vi "File_Create Linker files.vi"(7 "Run Data":T1={"Target Folder"=path "", "Menu Folder"=path "", "Active Folder"=path "", "Config"={"Main"={"Menu Folder"="", "Re-Create Menu Folder?"=FALSE, "Allow mnu replace?"=FALSE, "Relative Link Target"=""}, "File Filter"={"Exclude Prefixes"=[], "Ignore Names"=[], "Include Extensions"=[], "Exclude Postfixes"=[]}, "Folder Filter"={"Exclude Prefixes"=[], "Ignore Names"=[]}, "File Name Edit"={"Pre Split String"="", "Post Split String"="", "Deletion Strings"=[]}, "Folder Name Edit"={"Pre Split String"="", "Post Split String"="", "Deletion Strings"=[]}, "Folder Icon Map"={}, "Default Palette Data"={"Display Name Override"="", "View Format"=2, "Palette Width"=0, "Help Tag"="", "Help File Path"=path "", "Palette Description"=""}, "Default File Data"={"Display Name Override"="", "Place VI Contents?"=FALSE}, "Palette Override map"={}, "File Override map"={}}} {"Config"."Default Palette Data"."View Format" items=["Icons", "Text", "Icons and Text"]}, 8 "error in (no error)":errorcluster, 10 "Link Target Root Override (\"\")":path, 11 "Created mnu file paths":path[](array[path])) -> (0 "error out":errorcluster, 1 "Link files created?":bool, 2 "Unlinker":path, 3 "Linker":path)   [LabVIEW 2019, in "AutoMenuCreator.lvlib"]
uses:
  AutoMenuCreator.lvlib
  Ctl/Ctl_Run Data.ctl
  Ctl/Ctl_Config.ctl
  Ctl/Ctl_Config_Main.ctl
  Ctl/Ctl_Config_File Filter.ctl
  Ctl/Ctl_Config_Folder Filter.ctl
  Ctl/Ctl_Config_Name Edit.ctl
  Ctl/Ctl_Config_Folder Icon Map.ctl
  Ctl/Ctl_Config_Palette Data.ctl
  <vilib>/Palette API/Palette Menu/Public Type Define/View Format.ctl
  Ctl/Ctl_Config_File Data.ctl
  <vilib>/Palette API/Palette Menu/Palette Menu.lvlib
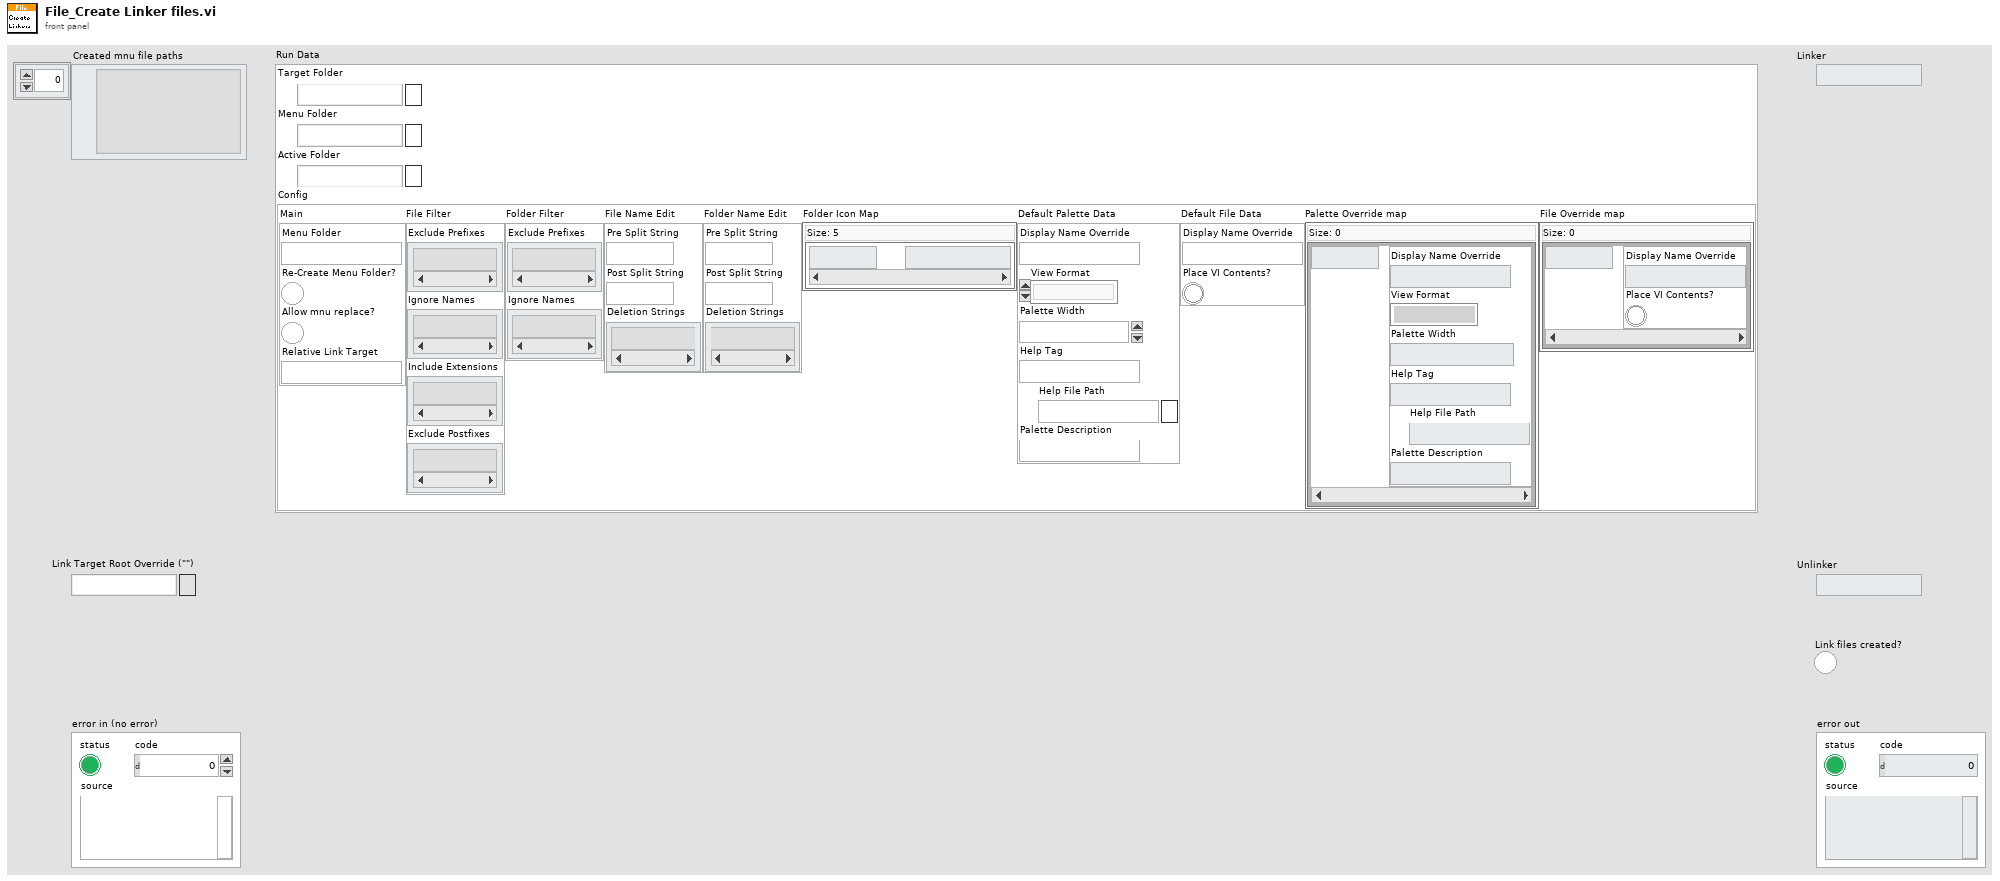
[diagram p1: front panel]
types:
  T1 = typedef "AutoMenuCreator.lvlib/Ctl_Run Data.ctl" = cluster{"Target Folder":path, "Menu Folder":path, "Active Folder":path, "Config":T2}
  T2 = typedef "AutoMenuCreator.lvlib/Ctl_Config.ctl" = cluster{"Main":T3, "File Filter":T4, "Folder Filter":T5, "File Name Edit":T6, "Folder Name Edit":T6, "Folder Icon Map":T7, "Default Palette Data":T8, "Default File Data":T10, "Palette Override map":map{string, T8}, "File Override map":map{string, T10}}
  T3 = typedef "AutoMenuCreator.lvlib/Ctl_Config_Main.ctl" = cluster{"Menu Folder":string, "Re-Create Menu Folder?":bool, "Allow mnu replace?":bool, "Relative Link Target":string}
  T4 = typedef "AutoMenuCreator.lvlib/Ctl_Config_File Filter.ctl" = cluster{"Exclude Prefixes":string[], "Ignore Names":string[], "Include Extensions":string[], "Exclude Postfixes":string[]}
  T5 = typedef "AutoMenuCreator.lvlib/Ctl_Config_Folder Filter.ctl" = cluster{"Exclude Prefixes":string[], "Ignore Names":string[]}
  T6 = typedef "AutoMenuCreator.lvlib/Ctl_Config_Name Edit.ctl" = cluster{"Pre Split String":string, "Post Split String":string, "Deletion Strings":string[]}
  T7 = typedef "AutoMenuCreator.lvlib/Ctl_Config_Folder Icon Map.ctl" = map{string, path}
  T8 = typedef "AutoMenuCreator.lvlib/Ctl_Config_Palette Data.ctl" = cluster{"Display Name Override":string, "View Format":T9, "Palette Width":i16, "Help Tag":string, "Help File Path":path, "Palette Description":string}
  T9 = typedef "Palette Menu.lvlib/View Format.ctl" = u16
  T10 = typedef "AutoMenuCreator.lvlib/Ctl_Config_File Data.ctl" = cluster{"Display Name Override":string, "Place VI Contents?":bool}
  T11 = enum16{"open", "replace", "create", "open or create", "replace or create", "replace or create with confirmation"}
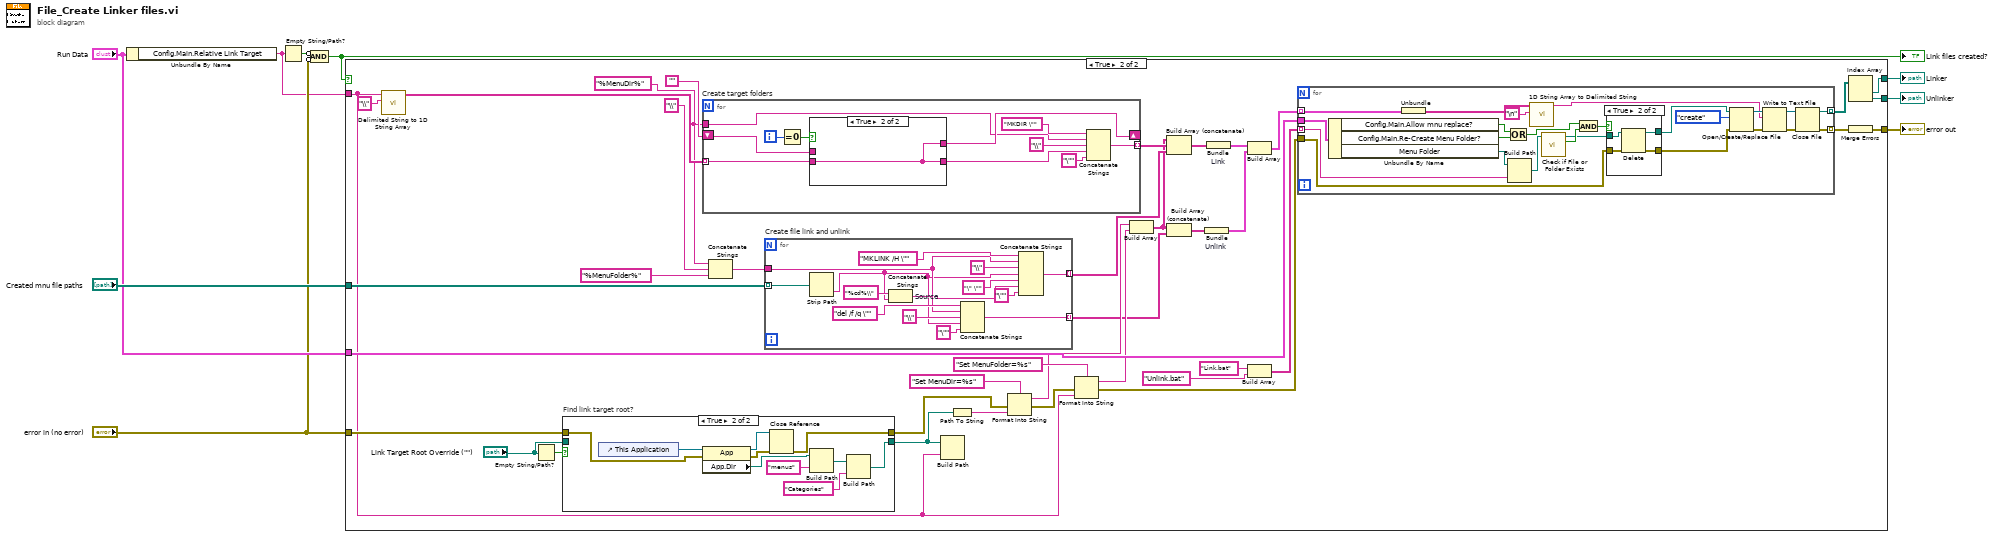
[diagram p0: block diagram]
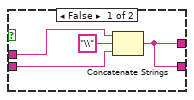
[diagram p4: hidden frame]
diagram:
  n1 = Unbundle By Name("Run Data") -> ("Config.Main.Relative Link Target"=w4:string)
  n2 = Empty String/Path?(string/path=w4) -> (empty?=w7:bool)
  n3 = Compound Arithmetic op=AND(invert w7, invert "error in (no error)") -> (w5:bool)
  "Link files created?" <- w5
  n4 = case shown="True" w5 {
    tunnel: "Created mnu file paths" -> [_ w49]
    tunnel: "Run Data" -> [_ w33]
    tunnel: "error in (no error)" -> [w10 w46]
    tunnel: w4 -> [_ w23]
    tunnel: [w10 w31] -> w3
    tunnel: [_ w29] -> w2
    tunnel: [_ w28] -> w1
    frame False {
    }
    frame True {
      w13 = "%MenuDir%"
      n5 = call <vilib>:"Delimited String to 1D String Array.vi"("delimiter"="\\", "delimited string"=w23) -> ("string array"=w44:string[])  [unwired: 9 in]
      n6 = Empty String/Path?(string/path="Link Target Root Override (\"\")") -> (empty?=w48:bool)
      n7 = case "Find link target root?" shown="True" w48 {
        tunnel: [w97 w100] -> w27
        tunnel: "Link Target Root Override (\"\")" -> [w97 _]
        tunnel: w46 -> [w96 w99]
        tunnel: [w96 w98] -> w21
        frame False {
        }
        frame True {
          n8 = control-ref of="This Application"() -> (w107:refnum<vi>)
          n9 = property class="App"(reference=w107, error in=w99) -> (reference out=w105:refnum<vi>, error out=w106:errorcluster, "App.Dir"=w104:path)
          n10 = Close Reference(reference=w105, error in (no error)=w106) -> (error out=w98:errorcluster)
          n11 = Build Path(base path=w104, name or relative path="menus") -> (appended path=w102:path)
          n12 = Build Path(base path=w102, name or relative path="Categories") -> (appended path=w100:path)
        }
      }
      n13 = for "Create target folders" {
        tunnel: w44 -> [w88] mode=indexing
        shift-right: [w86] -> _
        shift-left: "" -> [w87]
        tunnel: [w80] -> w42 mode=indexing
        tunnel: w13 -> [w84]
        i -> [w90]
        n14 = Equal To 0?(x=w90) -> (x = 0?=w89:bool)
        n15 = case shown="True" w89 {
          tunnel: [w91 w95] -> w82
          tunnel: w88 -> [w92 w95]
          tunnel: w87 -> [w94 _]
          tunnel: [w91 w95] -> w86
          frame False {
            n16 = Concatenate Strings(w94, "\\" ("string"), w92) -> (w91:string)
          }
          frame True {
          }
        }
        n17 = Concatenate Strings("MKDIR \"" ("string"), w84, "\\" ("string"), w82, "\"" ("string")) -> (w80:string)
      }
      n18 = Concatenate Strings(w13, "\\" ("string"), "%MenuFolder%") -> (w19:string)
      n19 = for "Create file link and unlink" {
        tunnel: w49 -> [w121] mode=indexing
        tunnel: [w109] -> w41 mode=indexing
        tunnel: [w116] -> w15 mode=indexing
        tunnel: w19 -> [w114]
        n20 = Strip Path(path=w121) -> (name=w108:string)  [unwired: 1 out]
        n21 = Concatenate Strings "Source"("%cd%\\", w108) -> (w111:string)
        n22 = Concatenate Strings("del /f /q \"" ("string"), w114, "\\" ("string"), w108, "\"" ("string")) -> (w116:string)
        n23 = Concatenate Strings("MKLINK /H \"" ("string"), w114, "\\" ("string"), w108, "\" \"" ("string"), w111, "\"" ("string")) -> (w109:string)
      }
      n24 = Build Path(base path=w27, name or relative path=w23) -> ()  [unwired: 1 out]
      n25 = Path To String(path=w27) -> (string=w25:string)
      n26 = Format Into String(format string="Set MenuDir=%s", error in=w21, w25) -> (resulting string=w18:string, error out=w22:errorcluster)  [unwired: 1 in]
      n27 = Format Into String(format string="Set MenuFolder=%s", error in=w22, w23) -> (resulting string=w17:string, error out=w11:errorcluster)  [unwired: 1 in]
      n28 = Build Array(w18, w17) -> (w16:string[])
      n29 = Build Array (concatenate)(w16, w42, w41) -> (w40:string[])
      n30 = Build Array (concatenate)(w16, w15) -> (w14:string[])
      n31 = Bundle "Unlink"(w14) -> (w38:cluster{string[]})  [unwired: 1 in]
      n32 = Bundle "Link"(w40) -> (w39:cluster{string[]})  [unwired: 1 in]
      n33 = Build Array(w39, w38) -> (w37:cluster{string[]}[])
      n34 = Build Array("Link.bat" ("string"), "Unlink.bat" ("string")) -> (w34:string[])
      n35 = for {
        tunnel: w11 -> [w63]
        tunnel: w37 -> [w73] mode=indexing
        tunnel: w34 -> [w68] mode=indexing
        tunnel: w33 -> [w71]
        tunnel: [w51] -> w32 mode=indexing
        tunnel: [w50] -> w30 mode=indexing
        n36 = Unbundle By Name(w71) -> ("Config.Main.Allow mnu replace?"=w70:bool, "Config.Main.Re-Create Menu Folder?"=w72:bool, "Menu Folder"=w69:path)
        n37 = Unbundle(w73) -> (w58:string[])
        n38 = Or(x=w70, y=w72) -> (x .or. y?=w65:bool)
        n39 = Build Path(base path=w69, name or relative path=w68) -> (appended path=w67:path)
        n40 = call <vilib>:"1D String Array to Delimited String.vi"("delimiter"="\n", "string array"=w58) -> ("delimited string"=w55:string)  [unwired: 9 in]
        n41 = call <vilib>:"Check if File or Folder Exists.vi"("path"=w67) -> ("file or folder exists?"=w66:bool, "dup path"=w62:path)  [unwired: 8 in, 1 out]
        n42 = And(x=w65, y=w66) -> (x .and. y?=w64:bool)
        n43 = case shown="True" w64 {
          tunnel: [w75 w78] -> w59
          tunnel: w63 -> [w75 w79]
          tunnel: w62 -> [w74 w77]
          tunnel: [w74 w76] -> w61
          frame False {
          }
          frame True {
            n44 = Delete(path (use dialog)=w77, error in=w79) -> (deleted path=w76:path, error out=w78:errorcluster)  [unwired: 3 in, 1 out]
          }
        }
        n45 = Open/Create/Replace File(file path (use dialog)=w61, error in=w59, operation (0:open)=T11."create") -> (refnum out=w56:refnum<file>, error out=w54:errorcluster)  [unwired: 3 in, 1 out]
        n46 = Write to Text File(file (use dialog)=w56, text=w55, error in=w54) -> (refnum out=w53:refnum<file>, error out=w52:errorcluster)  [unwired: 1 in, 1 out]
        n47 = Close File(refnum=w53, error in=w52) -> (path=w50:path, error out=w51:errorcluster)
      }
      n48 = Index Array(array=w30) -> (element #1=w29:path, element #2=w28:path)  [unwired: 2 in]
      n49 = Merge Errors(w32) -> (w31:errorcluster)
    }
  }
  "error out" <- w3
  "Linker" <- w2
  "Unlinker" <- w1
